vi "LabVIEW project.vi"() -> ()   [LabVIEW 2019]
uses:
  <vilib>/myRIO/Instrument Drivers/Onboard IO/SPI/typedefs/SPI User Configuration.ctl
  <vilib>/myRIO/Common/Instrument Driver Framework/myRIO v1.0/SPI/typedefs/SPI Clock Phase.ctl
  <vilib>/myRIO/Common/Instrument Driver Framework/myRIO v1.0/SPI/typedefs/SPI Clock Polarity.ctl
  <vilib>/myRIO/Common/Instrument Driver Framework/myRIO v1.0/SPI/typedefs/SPI Data Direction.ctl
  <vilib>/myRIO/Common/Instrument Driver Framework/myRIO v1.0/SPI/typedefs/SPI Frame Length.ctl
  <vilib>/myRIO/Common/Instrument Driver Framework/myRIO v1.0/DIO/vis/myRIO v1.1 Open DIO.vi
  <vilib>/myRIO/Common/Instrument Driver Framework/myRIO v1.0/SPI/vis/myRIO v1.1 Open SPI.vi
  <vilib>/myRIO/Instrument Drivers/Onboard IO/SPI/vis/Write Read.vi
  <vilib>/myRIO/Common/Instrument Driver Framework/myRIO v1.0/UART/vis/myRIO v1.0 Close UART.vi
  <vilib>/myRIO/Common/Instrument Driver Framework/Utilities/vis/Validate Channels.vi
  <vilib>/myRIO/Common/Instrument Driver Framework/myRIO v1.0/DIO/vis/myRIO v1.0 Reserve DIO.vi
  <vilib>/myRIO/Common/Instrument Driver Framework/myRIO v1.0/SPI/vis/myRIO v1.0 Reserve SPI.vi
  <vilib>/myRIO/Common/Instrument Driver Framework/myRIO v1.0/Resource Manager/vis/myRIO v1.0 Reserve Channel List.vi
  <vilib>/myRIO/Common/Instrument Driver Framework/myRIO v1.0/DIO/vis/myRIO v1.0 Build MUX Configuration DIO.vi
  <vilib>/myRIO/Common/Instrument Driver Framework/myRIO v1.0/SPI/vis/myRIO v1.0 Build MUX Configuration SPI.vi
  <vilib>/myRIO/Common/Instrument Driver Framework/myRIO v1.0/Resource Manager/vis/myRIO v1.0 Reserve Channel.vi
  <vilib>/myRIO/Common/Instrument Driver Framework/myRIO v1.0/Resource Manager/vis/myRIO v1.0 Unreserve Channel.vi
  <vilib>/myRIO/Common/Instrument Driver Framework/myRIO v1.0/Resource Manager/vis/myRIO v1.0 Create Configuration List.vi
  <vilib>/myRIO/Common/Instrument Driver Framework/myRIO v1.0/Resource Manager/vis/myRIO v1.0 Build Mutex Name.vi
  <vilib>/Utility/VariantDataType/GetNumericInfo.vi
  <vilib>/Utility/error.llb/Error Cluster From Error Code.vi
  <vilib>/myRIO/Common/Instrument Driver Framework/myRIO v1.0/myRIO v1.1 Open.vi
  <vilib>/myRIO/Common/Instrument Driver Framework/Utilities/vis/IO Manager.vi
  <vilib>/myRIO/Common/Instrument Driver Framework/Utilities/vis/Configuration Manager.vi
  <vilib>/myRIO/Common/Instrument Driver Framework/myRIO v1.0/Resource Manager/vis/myRIO v1.0 Configure IO.vi
  <vilib>/myRIO/Common/Instrument Driver Framework/myRIO v1.0/myRIO v1.0 Close.vi
  <vilib>/myRIO/Common/Instrument Driver Framework/myRIO v1.0/SPI/vis/myRIO v1.0 Configure SPI.vi
  <vilib>/myRIO/Common/Instrument Driver Framework/myRIO v1.0/DIO/vis/myRIO v1.0 Write DIO.vi
  <vilib>/myRIO/Common/Instrument Driver Framework/myRIO v1.0/SPI/vis/myRIO v1.0 Write Read SPI.vi
  <vilib>/myRIO/Common/Instrument Driver Framework/Utilities/vis/FPGA Ref Manager.vi
  <vilib>/myRIO/Common/Instrument Driver Framework/myRIO v1.0/myRIO v1.0 Reset FPGA.vi
  <vilib>/myRIO/Common/Instrument Driver Framework/myRIO v1.0/IRQ/vis/myRIO v1.0 IRQ Info FGV.vi
  <vilib>/myRIO/Common/Instrument Driver Framework/myRIO v1.0/IRQ/vis/myRIO v1.0 Timer IRQ Info FGV.vi
  <vilib>/myRIO/Common/Instrument Driver Framework/myRIO v1.0/IRQ/vis/myRIO v1.0 ISR Agent.vi
  <vilib>/myRIO/Instrument Drivers/Utilities/vis/Reset Index.vi
  <vilib>/myRIO/Common/Instrument Driver Framework/myRIO v1.0/Resource Manager/vis/myRIO v1.0 Block Write Resource Manager.vi
  <vilib>/myRIO/Instrument Drivers/Onboard IO/SPI/SPI.lvlib
  <vilib>/myRIO/Instrument Drivers/Onboard IO/DIO/DIO.lvlib
  <vilib>/myRIO/Instrument Drivers/Utilities/Utilities.lvlib
panel:
  in  "stop":bool
  out "Graph":dbl(graph)
  in  "Amplitude":dbl
  in  "Phase (in degrees)":dbl
  in  "Frequency (in Hz)":dbl
  in  "Select Save":bool
  in  "Save":bool
  in  "Starting address":u16 max=511 step=1 format="%0d"
  out "EEPROM array":u16[](array[numeric]) format="%0d"
  in  "ESC":bool
  in  "Write protect":bool=TRUE
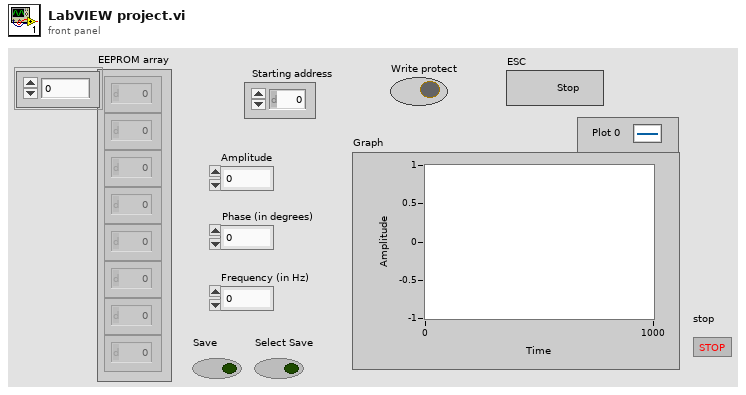
[diagram p1: front panel]
types:
  T1 = typedef "SPI.lvlib/SPI User Configuration.ctl" = cluster{"Frequency [Hz]":dbl, "Clock Phase":T2, "Clock Polarity":T3, "Data Direction":T4, "Frame Length":T5}
  T2 = typedef "SPI Clock Phase.ctl" = enum8{"Leading", "Trailing"}
  T3 = typedef "SPI Clock Polarity.ctl" = enum8{"Low", "High"}
  T4 = typedef "SPI Data Direction.ctl" = enum8{"Most significant bit first", "Least significant bit first"}
  T5 = typedef "SPI Frame Length.ctl" = u8
  T6 = typedef "DIO.lvlib/DIO Reference.ctl" = cluster{"myRIO Reference":T7, "DIO Channels List":T11}
  T7 = typedef "myRIO Generic Hardware Reference.ctl" = cluster{"myRIO Model":T8, "myRIO Hardware Reference":T9}
  T8 = typedef "Hardware Version Enum.ctl" = enum16{"Unknown", "myRIO-1900", "myRIO-1950", "roboRIO", "NI ELVIS RIO CM", "ELVIS III"}
  T9 = typedef "myRIO v1.0 Reference.ctl" = cluster{"Generic FPGA Reference":T10, "Allow multiple opens":bool}
  T10 = typedef "Generic FPGA Reference.ctl" = refnum<k20>
  T11 = typedef "DIO Channels List.ctl" = T12[]
  T12 = typedef "DIO Channels Enum.ctl" = enum16{"Not Connected", "C/DIO0", "C/DIO1", "C/DIO2", "C/DIO3", "C/DIO4", "C/DIO5", "C/DIO6", "C/DIO7", "A/DIO0", "A/DIO1", "A/DIO2", "A/DIO3", "A/DIO4", "A/DIO5", "A/DIO6", "A/DIO7", "A/DIO8", "A/DIO9", "A/DIO10", "A/DIO11", "A/DIO12", "A/DIO13", "A/DIO14", "A/DIO15", "A/DIO16", "A/DIO17", "A/DIO18", "A/DIO19", "B/DIO0", "B/DIO1", "B/DIO2", "B/DIO3", "B/DIO4", "B/DIO5", "B/DIO6", "B/DIO7", "B/DIO8", "B/DIO9", "B/DIO10", "B/DIO11", "B/DIO12", "B/DIO13", "B/DIO14", "B/DIO15", "B/DIO16", "B/DIO17", "B/DIO18", "B/DIO19", "LED0", "LED1", "LED2", "LED3", "Button0", "DIO/DIO0", "DIO/DIO1", "DIO/DIO2", "DIO/DIO3", "DIO/DIO4", "DIO/DIO5", "DIO/DIO6", "DIO/DIO7", "DIO/DIO8", "DIO/DIO9", "SPI/CS0", "SPI/CS1", "SPI/CS2", "SPI/CS3", "LED RADIO (Green)", "LED RADIO (Red)", "LED COMM (Green)", "LED COMM (Red)", "LED MODE (Green)", "LED MODE (Red)"}
  T13 = typedef "SPI.lvlib/SPI Reference.ctl" = cluster{"myRIO Reference":T7, "SPI Channels Enum":T14, "SPI Configuration":T15}
  T14 = typedef "SPI Channels Enum.ctl" = enum16{"Not Connected", "A/SPI", "B/SPI", "SPI/SPI"}
  T15 = typedef "SPI.lvlib/SPI Configuration.ctl" = cluster{"Frequency [Hz]":dbl, "Clock Phase":T2, "Clock Polarity":T3, "Data Direction":T4, "Frame Length":T5}
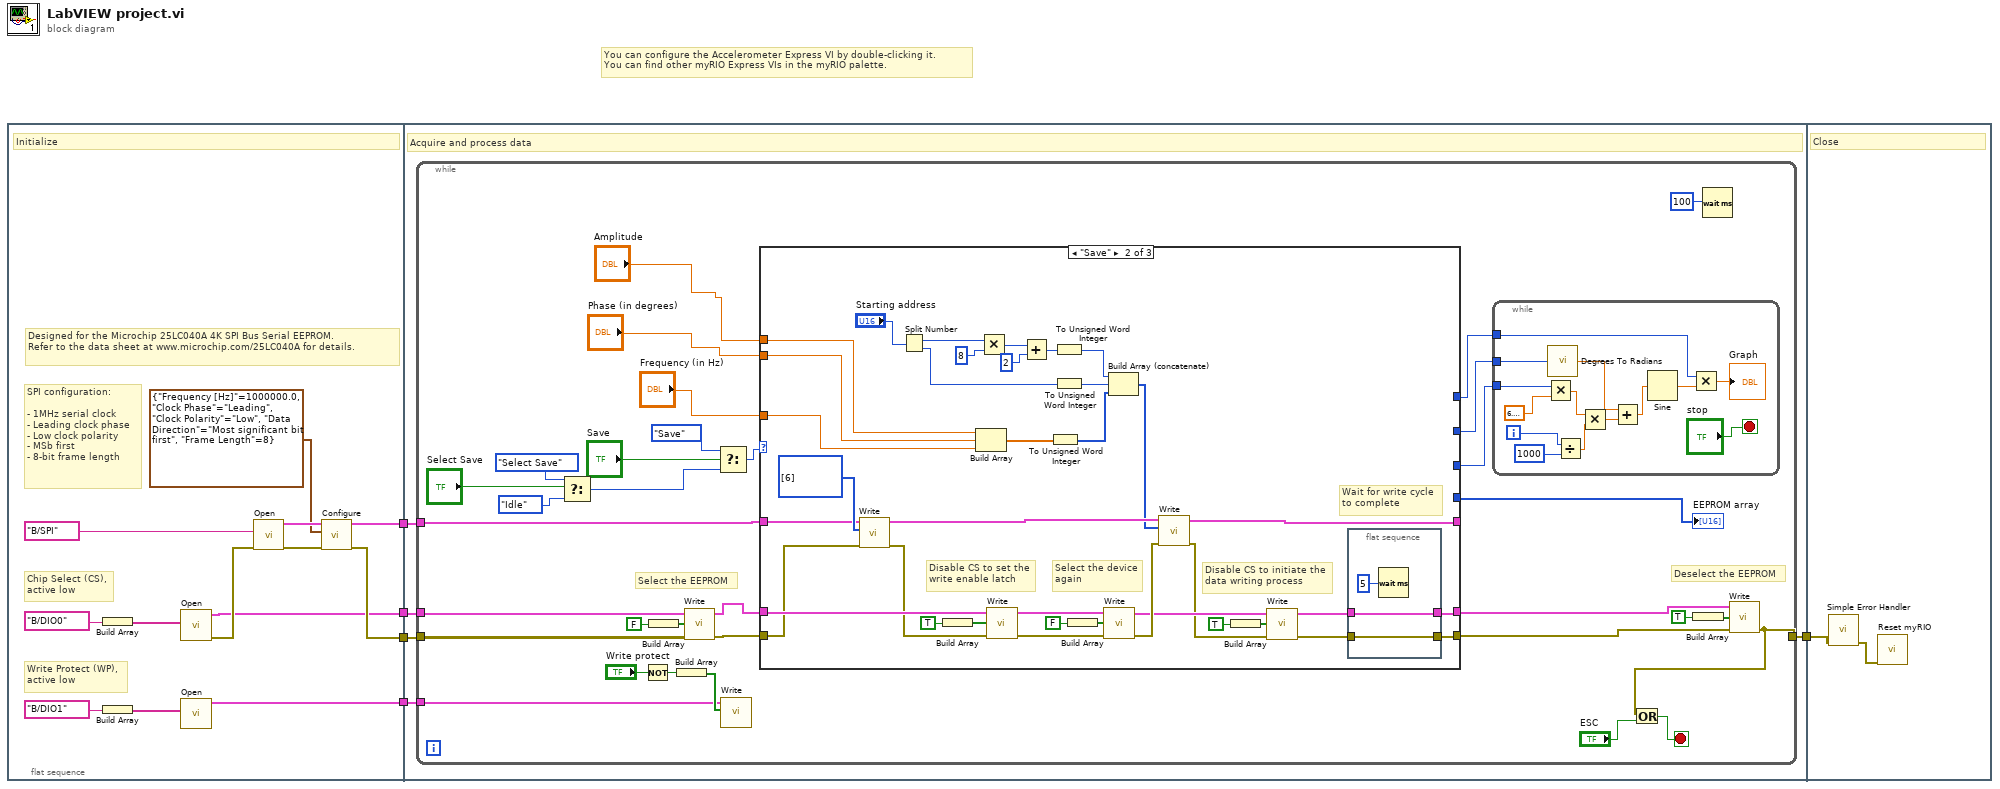
[diagram p0: block diagram]
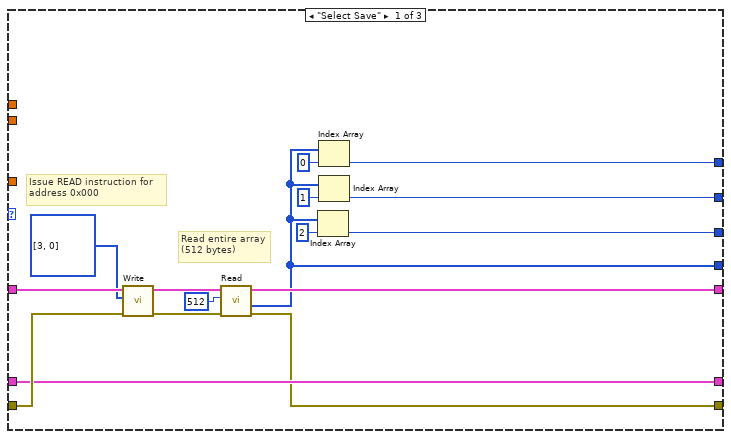
[diagram p2: hidden frame]
diagram:
  # "You can configure the Accelerometer Express VI by double-clicking it.\nYou can find other myRIO Express VIs in the myRIO palette."
  n1 = flat-sequence {
    tunnel: [w9] -> w5
    tunnel: [w8] -> w4
    tunnel: [w7] -> w3
    tunnel: [w6] -> w2
    tunnel: w5 -> [w23]
    tunnel: w4 -> [w22]
    tunnel: w3 -> [w21]
    tunnel: w2 -> [w20]
    tunnel: [w19] -> w1
    tunnel: w1 -> [w130]
    frame #0 {
      # "Write Protect (WP),\nactive low"
      # "Chip Select (CS),\nactive low"
      # "SPI configuration:\n\n- 1MHz serial clock\n- Leading clock phase\n- Low clock polarity\n- MSb first\n- 8-bit frame length"
      # "Designed for the Microchip 25LC040A 4K SPI Bus Serial EEPROM.\nRefer to the data sheet at www.microchip.com/25LC040A for details."
      # "Initialize"
      n2 = Build Array "Build Array"(tag "B/DIO0" ("myRIO DIO Channel")) -> (w17:tag[])
      n3 = Build Array(tag "B/DIO1" ("myRIO DIO Channel")) -> (w18:tag[])
      n4 = call <vilib>:"Open.vi"("Channel Names"=w17) -> ("error out"=w16:errorcluster, "DIO Ref Out"=w6:T6)  [unwired: 9 in]
      n5 = call <vilib>:"Open.vi"("Channel Names"=w18) -> ("DIO Ref Out"=w7:T6)  [unwired: 9 in, 1 out]
      n6 = call <vilib>:"Open.vi"("error in (no error)"=w16, "Channel Name"=tag "B/SPI") -> ("error out"=w15:errorcluster, "SPI Ref Out"=w14:T13)  [unwired: 8 in]
      n7 = call <vilib>:"Configure.vi"("error in (no error)"=w15, "SPI User Configuration"=T1 {"Frequency [Hz]"=1000000.0, "Clock Phase"=enum."Leading", "Clock Polarity"=enum."Low", "Data Direction"=enum."Most significant bit first", "Frame Length"=8}, "SPI Ref In"=w14) -> ("error out"=w9:errorcluster, "SPI Ref Out"=w8:T13)  [unwired: 7 in]
    }
    frame #1 {
      # "Acquire and process data"
      n8 = while {
        tunnel: w22 -> [w35]
        tunnel: w23 -> [w56]
        tunnel: [w37] -> w19
        tunnel: w21 -> [w49]
        tunnel: w20 -> [w40]
        stop <- w51 stop-if-true
        # "Deselect the EEPROM"
        # "Select the EEPROM"
        n9 = Select(t=enum16{"Idle", "Select Save", "Save"}."Select Save", s="Select Save", f=enum16{"Idle", "Select Save", "Save"}."Idle") -> (s? t:f=w45:enum16{"Idle", "Select Save", "Save"})
        n10 = Not(x="Write protect") -> (.not. x?=w55:bool)
        n11 = Build Array(FALSE) -> (w42:bool[])
        n12 = Build Array(w55) -> (w53:bool[])
        n13 = call <vilib>:"Write.vi"("error in (no error)"=w56, "Values"=w42, "DIO Ref In"=w40) -> ("error out"=w34:errorcluster, "DIO Ref Out"=w33:T6)  [unwired: 6 in]
        n14 = Select(t=enum16{"Idle", "Select Save", "Save"}."Save", s="Save", f=w45) -> (s? t:f=w36:enum16{"Idle", "Select Save", "Save"})
        n15 = call <vilib>:"Write.vi"("Values"=w53, "DIO Ref In"=w49) -> ()  [unwired: 7 in, 2 out]
        n16 = case shown="\"Save\"" w36 {
          tunnel: w35 -> [w86 w107 w129]
          tunnel: w34 -> [w85 w94 w128]
          tunnel: [w80 w123 w129] -> _
          tunnel: [w78 w95 w128] -> w31
          tunnel: w33 -> [w83 w108 w127]
          tunnel: [w83 w97 w127] -> w30
          tunnel: [w77 _ _] -> w29
          tunnel: "Phase (in degrees)" -> [_ w89 _]
          tunnel: "Frequency (in Hz)" -> [_ w88 _]
          tunnel: "Amplitude" -> [_ w87 _]
          tunnel: [w73 _ _] -> w26
          tunnel: [w72 _ _] -> w25
          tunnel: [w71 _ _] -> w24
          frame "Select Save" {
            # "Read entire array\n(512 bytes)"
            # "Issue READ instruction for\naddress 0x000"
            n17 = call <vilib>:"Write.vi"("error in (no error)"=w85, "Frames to Write"=u16[] [3, 0], "SPI Ref In"=w86) -> ("error out"=w79:errorcluster, "SPI Ref Out"=w81:T13)  [unwired: 7 in]
            n18 = call <vilib>:"Read.vi"("error in (no error)"=w79, "Frame Count"=u32 512, "SPI Ref In"=w81) -> ("error out"=w78:errorcluster, "Frames Read"=w77:u16[], "SPI Ref Out"=w80:T13)  [unwired: 5 in]
            n19 = Index Array(array=w77, index=2) -> (element=w71:u16)
            n20 = Index Array(array=w77, index=0) -> (element=w73:u16)
            n21 = Index Array(array=w77, index=1) -> (element=w72:u16)
          }
          frame "Save" {
            # "Wait for write cycle\nto complete"
            # "Disable CS to initiate the\ndata writing process"
            # "Select the device\nagain"
            # "Disable CS to set the\nwrite enable latch"
            n22 = call <vilib>:"Write.vi"("error in (no error)"=w94, "Frames to Write"=u16[] [6], "SPI Ref In"=w107) -> ("error out"=w93:errorcluster, "SPI Ref Out"=w106:T13)  [unwired: 7 in]
            n23 = Split Number(x="Starting address") -> (hi(x)=w121:u8, lo(x)=w116:u8)
            n24 = Build Array(TRUE) -> (w112:bool[])
            n25 = Build Array "Build Array"(w87, w89, w88) -> (w92:dbl[])
            n26 = Multiply(x=w121, y=u8 8) -> (x*y=w119:u8)
            n27 = call <vilib>:"Write.vi"("error in (no error)"=w93, "Values"=w112, "DIO Ref In"=w108) -> ("error out"=w111:errorcluster, "DIO Ref Out"=w113:T6)  [unwired: 6 in]
            n28 = Add(x=w119, y=u8 2) -> (x+y=w117:u8)
            n29 = To Unsigned Word Integer(number=w92) -> (unsigned 16bit integer=w91:u16[])
            n30 = To Unsigned Word Integer(number=w117) -> (unsigned 16bit integer=w115:u16)
            n31 = To Unsigned Word Integer(number=w116) -> (unsigned 16bit integer=w114:u16)
            n32 = Build Array(FALSE) -> (w103:bool[])
            n33 = call <vilib>:"Write.vi"("error in (no error)"=w111, "Values"=w103, "DIO Ref In"=w113) -> ("error out"=w105:errorcluster, "DIO Ref Out"=w100:T6)  [unwired: 6 in]
            n34 = Build Array (concatenate) "Build Array"(w115, w114, w91) -> (w90:u16[])
            n35 = call <vilib>:"Write.vi"("error in (no error)"=w105, "Frames to Write"=w90, "SPI Ref In"=w106) -> ("error out"=w99:errorcluster, "SPI Ref Out"=w123:T13)  [unwired: 7 in]
            n36 = Build Array(TRUE) -> (w101:bool[])
            n37 = call <vilib>:"Write.vi"("error in (no error)"=w99, "Values"=w101, "DIO Ref In"=w100) -> ("error out"=w96:errorcluster, "DIO Ref Out"=w98:T6)  [unwired: 6 in]
            n38 = flat-sequence {
              tunnel: w98 -> [w125]
              tunnel: [w125] -> w97
              tunnel: w96 -> [w124]
              tunnel: [w124] -> w95
              frame #0 {
                n39 = Wait (ms)(milliseconds to wait=u32 5) -> ()  [unwired: 1 out]
              }
            }
          }
          frame "Idle", Default {
          }
        }
        "EEPROM array" <- w29
        n40 = while {
          tunnel: w24 -> [w60]
          tunnel: w25 -> [w59]
          tunnel: w26 -> [w58]
          i -> [w64]
          stop <- "stop" stop-if-true
          n41 = Multiply(x=w60, y=6.283185307179586) -> (x*y=w68:dbl)
          n42 = call "Degrees To Radians.vi"("Phase (in degrees)"=w59) -> ("Phase (in radians)"=w63:dbl)
          n43 = Divide(x=w64, y=1000) -> (x/y=w62:dbl)
          n44 = Multiply(x=w68, y=w62) -> (x*y=w67:dbl)
          n45 = Add(x=w63, y=w67) -> (x+y=w66:dbl)
          n46 = Sine(x=w66) -> (sin(x)=w70:dbl)
          n47 = Multiply(x=w58, y=w70) -> (x*y=→"Graph":dbl)
        }
        n48 = Build Array(TRUE) -> (w39:bool[])
        n49 = Wait (ms)(milliseconds to wait=u32 100) -> ()  [unwired: 1 out]
        n50 = call <vilib>:"Write.vi"("error in (no error)"=w31, "Values"=w39, "DIO Ref In"=w30) -> ("error out"=w37:errorcluster)  [unwired: 6 in, 1 out]
        n51 = Or(x=w37, y="ESC") -> (x .or. y?=w51:bool)
      }
    }
    frame #2 {
      # "Close"
      n52 = call <vilib>:"Simple Error Handler.vi"("error in (no error)"=w130) -> ("error out"=w131:errorcluster)  [unwired: 4 in, 4 out]
      n53 = call <vilib>:"Reset myRIO.vi"("error in (no error)"=w131) -> ()  [unwired: 10 in, 1 out]
    }
  }
